vi "Define.vi"(8 "error in":errorcluster, 9 "Address":i32[](array[numeric]), 10 "Node Refnum":refnum<k20>, 11 "Node in":refnum<class "Node.lvclass">) -> (0 "error out":errorcluster, 3 "Node out":refnum<class "Node.lvclass">)   [LabVIEW 2014, in "Node.lvclass"]
uses:
  Node.lvclass
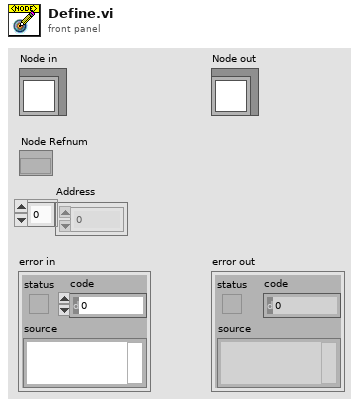
[diagram p1: front panel]
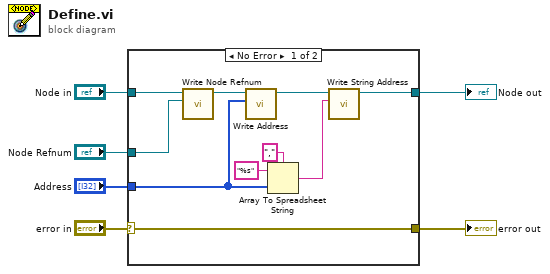
[diagram p0: block diagram]
diagram:
  n1 = case shown="No Error" "error in" {
    selector: "error in" -> [w16 w18]
    tunnel: [w16 w18] -> w5
    tunnel: [w10 w17] -> w4
    tunnel: "Node Refnum" -> [w13 _]
    tunnel: "Address" -> [w11 _]
    tunnel: "Node in" -> [w12 w17]
    frame No Error {
      n2 = call-dynamic "Write Node Refnum.vi"("Node Refnum"=w13, "Node in"=w12) -> ("Node out"=w15:refnum<class "Node.lvclass">)  [unwired: 8 in, 1 out]
      n3 = call-dynamic "Write Address.vi"("Address"=w11, "Node in"=w15) -> ("Node out"=w14:refnum<class "Node.lvclass">)  [unwired: 8 in, 1 out]
      n4 = Array To Spreadsheet String(delimiter (Tab)=",", array=w11, 3:"%s" ("format string")) -> (spreadsheet string=w8:string)
      n5 = call-dynamic "Write String Address.vi"("String Address"=w8, "Node in"=w14) -> ("Node out"=w10:refnum<class "Node.lvclass">)  [unwired: 8 in, 1 out]
    }
    frame Error {
    }
  }
  "error out" <- w5
  "Node out" <- w4
